vi "Compute DistanceToTarget2.vi"(9 "Long":bool, 10 "Norm Rect":T1, 11 "Camera Type":T2) -> (3 "Distance (ft)":dbl)   [LabVIEW 2014]
doc: "Using the camera lens information and the real world size of the target, use trig and ratios to determine the distance to the target. Also returns the location relative to the image center in a (-1 , 1) coordinate system that may be useful for steering the robot."
uses:
  2015 Dashboard Project/Camera Types.ctl
panel:
  # "Axis 206\nAxis M1011\nAxis M1013\nMS HD3000 square\nMS HD 3000 640x480"
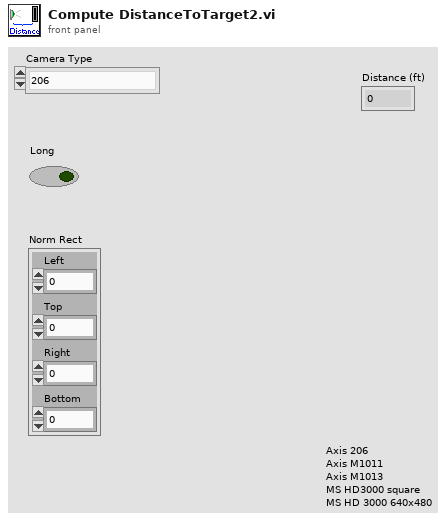
[diagram p1: front panel]
types:
  T1 = cluster{"Left":dbl, "Top":dbl, "Right":dbl, "Bottom":dbl}
  T2 = typedef "Camera Types.ctl" = enum16{"206", "1011", "1013", "MS HD3000 square", "MS HD3000 640x480"}
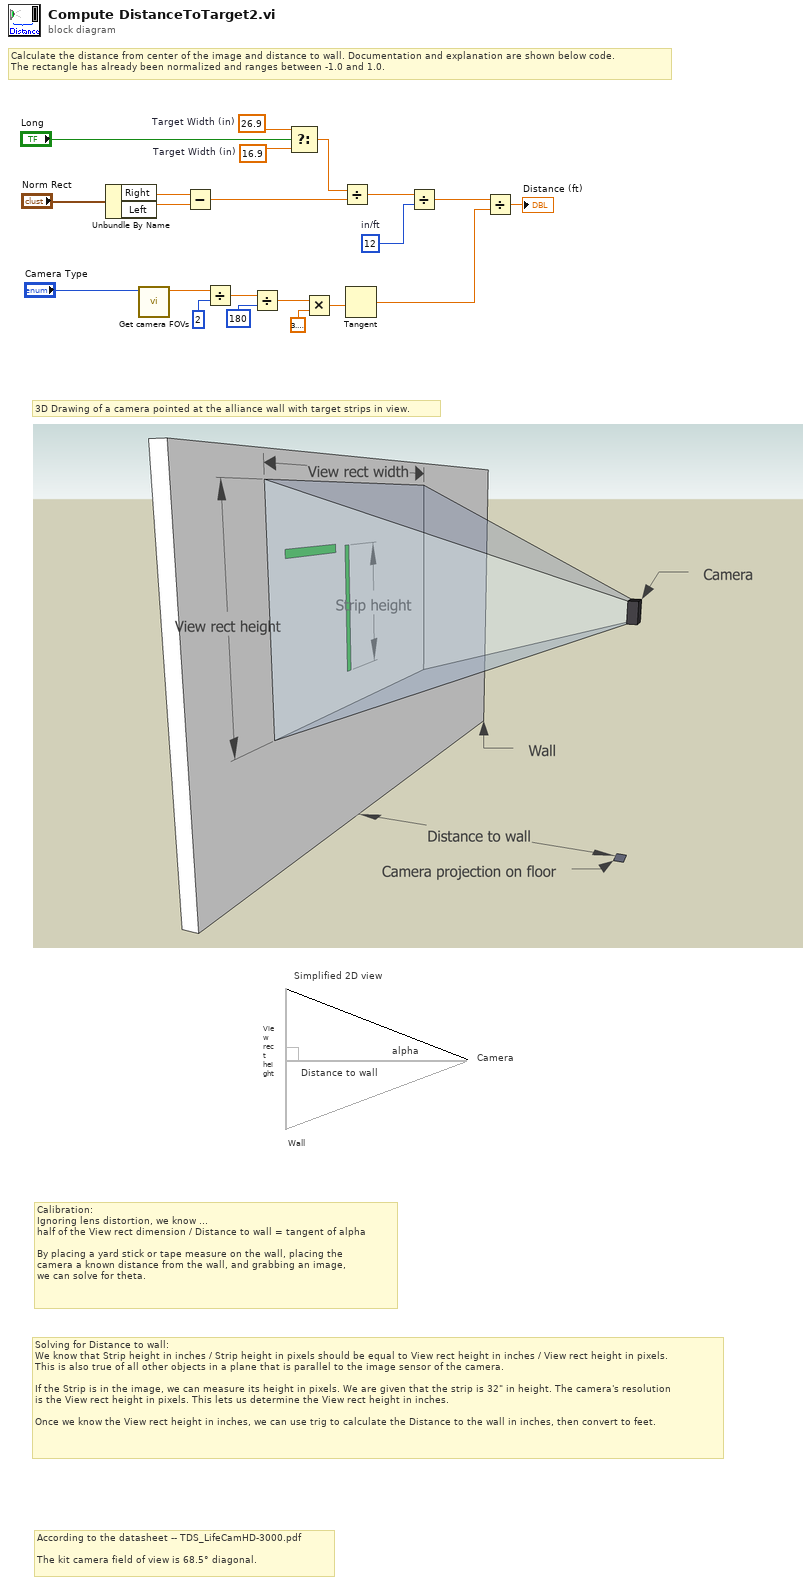
[diagram p0: block diagram]
diagram:
  w8 = 16.9  # Target Width (in)
  w9 = 26.9  # Target Width (in)
  w14 = 12  # in/ft
  # "According to the datasheet -- TDS_LifeCamHD-3000.pdf\n\nThe kit camera field of view is 68.5° diagonal."
  # "Wall"
  # "Camera"
  # "Simplified 2D view"
  # "Solving for Distance to wall:\nWe know that Strip height in inches / Strip height in pixels should be equal to View rect height in inches / View rect height in pixels.\nThis is also true of all other objects in a plane that is parallel to the image sensor of the camera.\n\nIf the Strip is in the image, we can measure its height in pixels. We are given that the strip is 32\" in height. The camera's resolution\nis the View rect height in pixels. This lets us determine the View rect height in inches.\n\nOnce we know the View rect height in inches, we can use trig to calculate the Distance to the wall in inches, then convert to feet."
  # "3D Drawing of a camera pointed at the alliance wall with target strips in view."
  # "Distance to wall"
  # "View rect height"
  # "alpha"
  # "Calibration:\nIgnoring lens distortion, we know ...\nhalf of the View rect dimension / Distance to wall = tangent of alpha\n\nBy placing a yard stick or tape measure on the wall, placing the\ncamera a known distance from the wall, and grabbing an image,\nwe can solve for theta."
  # "Calculate the distance from center of the image and distance to wall. Documentation and explanation are shown below code.\nThe rectangle has already been normalized and ranges between -1.0 and 1.0."
  n1 = Unbundle By Name("Norm Rect") -> ("Right"=w11:dbl, "Left"=w10:dbl)
  n2 = call "Get camera FOVs.vi"("Camera Type"="Camera Type") -> ("FOV"=w2:dbl)  [unwired: 9 in, 1 out]
  n3 = Subtract(x=w11, y=w10) -> (x-y=w5:dbl)
  n4 = Divide(x=w2, y=2) -> (x/y=w18:dbl)
  n5 = Divide(x=w18, y=180) -> (x/y=w17:dbl)
  n6 = Select(t=w9, s="Long", f=w8) -> (s? t:f=w7:dbl)
  n7 = Multiply(x=w17, y=3.141592653589793) -> (x*y=w19:dbl)
  n8 = Divide(x=w7, y=w5) -> (x/y=w4:dbl)
  n9 = Tangent(1:w19) -> (0:w13:dbl)
  n10 = Divide(x=w4, y=w14) -> (x/y=w3:dbl)
  n11 = Divide(x=w3, y=w13) -> (x/y=→"Distance (ft)":dbl)
